vi "Get All Tag Names from Table.vi"(8 "error in (no error)":errorcluster, 11 "Pairing Tab Refs":T1) -> (0 "error out":errorcluster, 2 "Tag Names":string[](array[string]))   [LabVIEW 2015, in "E2E Tag Exchange editor node.lvclass"]
uses:
  E2E Tag Exchange editor node.lvclass
  Tag Exchange Tab References.ctl
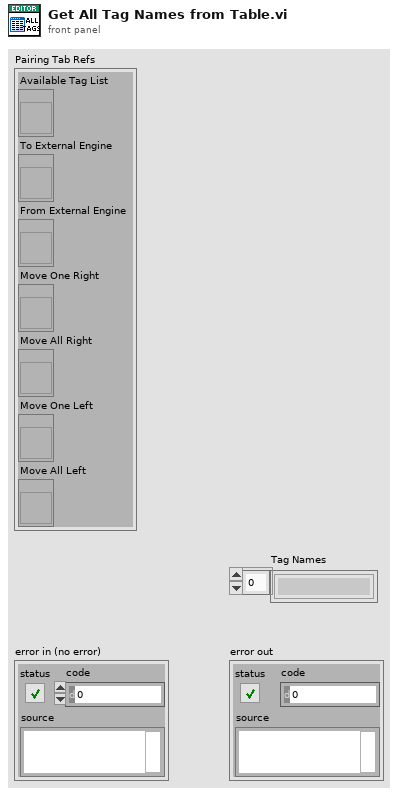
[diagram p1: front panel]
types:
  T1 = typedef "E2E Tag Exchange editor node.lvclass/Tag Exchange Tab References.ctl" = cluster{"Available Tag List":refnum<vi>, "To External Engine":refnum<vi>, "From External Engine":refnum<vi>, "Move One Right":refnum<vi>, "Move All Right":refnum<vi>, "Move One Left":refnum<vi>, "Move All Left":refnum<vi>}
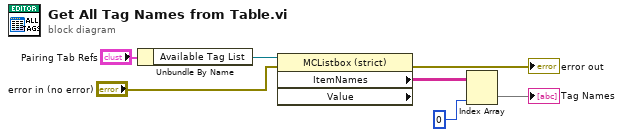
[diagram p0: block diagram]
diagram:
  n1 = Unbundle By Name("Pairing Tab Refs") -> ("Available Tag List"=w6:refnum<vi>)
  n2 = property class="MCListbox (strict)" props=["ItemNames", "Value"](reference=w6, error in="error in (no error)") -> (error out=→"error out":errorcluster, "ItemNames"=w5:string[][])  [unwired: 2 out]
  n3 = Index Array(array=w5, index (col)=0 ("disabled index (col)")) -> (element=→"Tag Names":string[])  [unwired: 1 in]
